vi "Read Analogue.vi"(8 "error in (no error)":errorcluster, 11 "Chroma 19020":refnum<class "Chroma 190020.lvclass">) -> (0 "error out":errorcluster, 2 "Waveforms":waveform(dbl)[](array[waveform]), 3 "Chroma 19020 out":refnum<class "Chroma 190020.lvclass">)   [LabVIEW 2025, in "HiPOT.lvlib" / "Chroma 190020.lvclass"]
uses:
  Chroma 190020.lvclass
  C:/Users/Public/Documents/Sandia National Labs/TSS Plugin/Abstract Engine.lvlibp/Abstract Instrument/Abstract Instrument.lvclass
  Chroma 190020.lvclass/Chroma 190020.ctl
  Read Index.vi
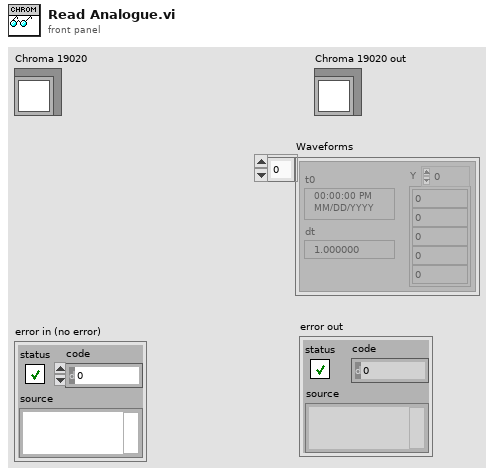
[diagram p1: front panel]
types:
  T1 = typedef "Abstract Engine.lvlibp/Abstract Instrument.lvclass/Channel.ctl" = cluster{"Alias":string, "DataType":enum16{"Anaolg Input", "Waveform"}, "Unit":enum16{"---", "V", "A", "Ohm", "Hz", "uF", "degC", "deg"}, "Upper limit":dbl, "Lower limit":dbl, "Measurement":variant}
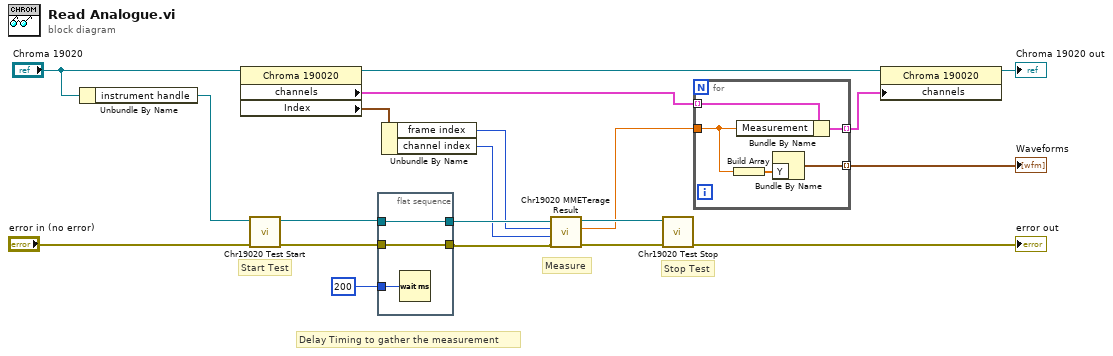
[diagram p0: block diagram]
diagram:
  # "Delay Timing to gather the measurement"
  # "Stop Test"
  # "Start Test"
  # "Measure"
  n1 = Unbundle By Name("Chroma 19020") -> ("instrument handle"=w12:refnum<k15>)
  n2 = property class="Chroma 190020"(reference="Chroma 19020") -> (reference out=w10:refnum<class "Chroma 190020.lvclass">, "channels"=w3:T1[], "Index"=w4:cluster{"frame index":i32, "channel index":i32})  [unwired: 1 in, 1 out]
  n3 = call <instrlib>:"Chr19020 Test Start.vi"("error in (no error)"="error in (no error)", "instrument handle"=w12) -> ("error out"=w17:errorcluster, "instrument handle out"=w18:refnum<k15>)  [unwired: 8 in]
  n4 = flat-sequence {
    tunnel: u32 200 -> [w21]
    tunnel: [w23] -> w7
    tunnel: w17 -> [w23]
    tunnel: [w22] -> w19
    tunnel: w18 -> [w22]
    frame #0 {
      n5 = Wait (ms)(milliseconds to wait=w21) -> ()  [unwired: 1 out]
    }
  }
  n6 = Unbundle By Name(w4) -> ("frame index"=w9:i32, "channel index"=w8:i32)
  n7 = call <instrlib>:"Chr19020 MMETerage Result.vi"("error in (no error)"=w7, "channel index"=w8, "frame index"=w9, "instrument handle"=w19) -> ("error out"=w15:errorcluster, "return value"=w5:dbl, "instrument handle out"=w16:refnum<k15>)  [unwired: 5 in]
  n8 = call <instrlib>:"Chr19020 Test Stop.vi"("error in (no error)"=w15, "instrument handle"=w16) -> ("error out"=→"error out":errorcluster)  [unwired: 8 in, 1 out]
  n9 = for {
    tunnel: w3 -> [w27] mode=indexing
    tunnel: [w28] -> w2 mode=indexing
    tunnel: w5 -> [w26]
    tunnel: [w24] -> w1 mode=indexing
    n10 = Build Array(w26) -> (w25:dbl[])
    n11 = Bundle By Name(cluster=w27, "Measurement"=w26) -> (w28:T1)
    n12 = Bundle By Name("Y"=w25) -> (w24:waveform(dbl))  [unwired: 1 in]
  }
  "Waveforms" <- w1
  n13 = property class="Chroma 190020"(reference=w10, "channels"=w2) -> (reference out=→"Chroma 19020 out":refnum<class "Chroma 190020.lvclass">)  [unwired: 1 in, 1 out]
